vi "Uniform_spaced_data.vi"(1 "Desired Times":dbl[](array[numeric]) format="%.2f", 2 "Eng Value":dbl[](array[numeric]) format="%.2f", 3 "Current Times":dbl[](array[numeric]) format="%.2f") -> (0 "Eng Values out":dbl[](array[numeric]) format="%.2f")   [LabVIEW 2010]
uses:
  <vilib>/Analysis/NI_AALPro.lvlib
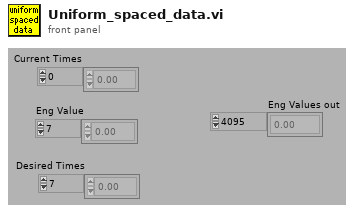
[diagram p1: front panel]
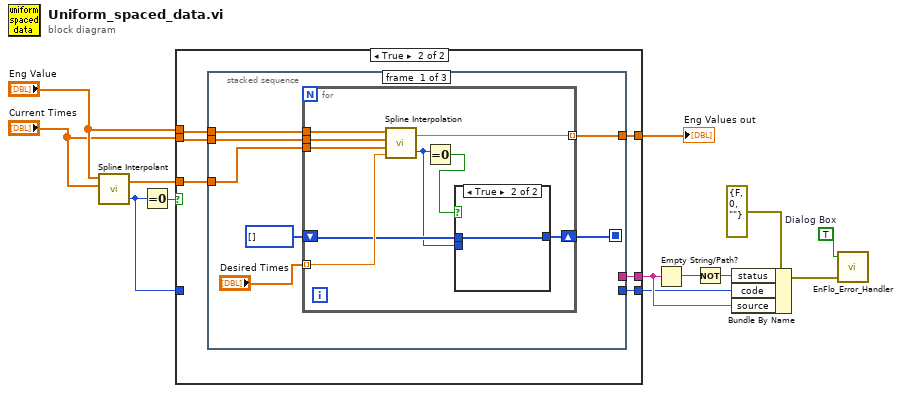
[diagram p0: block diagram]
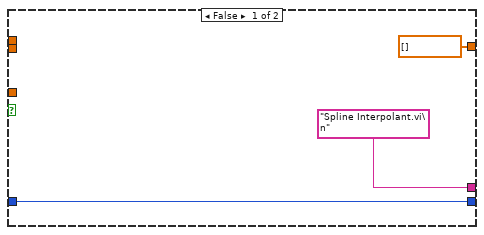
[diagram p2: hidden frame]
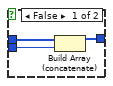
[diagram p3: hidden frame]
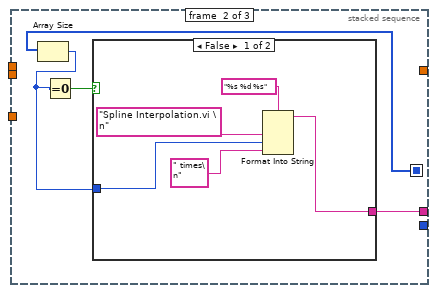
[diagram p4: hidden frame]
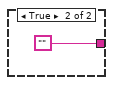
[diagram p5: hidden frame]
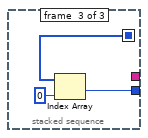
[diagram p6: hidden frame]
diagram:
  w2 = TRUE  # Dialog Box
  n1 = call <vilib>:"Spline Interpolant.vi"("X"="Current Times", "Y"="Eng Value") -> ("error"=w3:i32, "Interpolant"=w11:dbl[])  [unwired: 2 in]
  n2 = Equal To 0?(x=w3) -> (x = 0?=w8:bool)
  n3 = case shown="True" w8 {
    tunnel: "Eng Value" -> [_ w22]
    tunnel: "Current Times" -> [_ w21]
    tunnel: w11 -> [_ w20]
    tunnel: ["Spline Interpolant.vi\n" ("source") w19] -> w5
    tunnel: [w15 w18] -> w4
    tunnel: w3 -> [w15 _]
    tunnel: [dbl[] [] w17] -> w1
    frame False {
    }
    frame True {
      n4 = stacked-sequence {
        seq-local: [w24 _ _] -> [_ w43 w55]
        tunnel: w22 -> [w29 _ _]
        tunnel: w21 -> [w28 _ _]
        tunnel: w20 -> [w27 _ _]
        tunnel: [_ w44 _] -> w19
        tunnel: [_ _ w53] -> w18
        tunnel: [w23 _ _] -> w17
        frame #0 {
          n5 = for {
            tunnel: w29 -> [w38]
            tunnel: w28 -> [w37]
            tunnel: w27 -> [w36]
            tunnel: "Desired Times" -> [w35] mode=indexing
            shift-right: [w32] -> w24
            shift-left: i32[] [] -> [w33]
            tunnel: [w30] -> w23 mode=indexing
            n6 = call <vilib>:"Spline Interpolation.vi"("x value"=w35, "Interpolant"=w36, "X"=w37, "Y"=w38) -> ("error"=w31:i32, "interpolation value"=w30:dbl)
            n7 = Equal To 0?(x=w31) -> (x = 0?=w34:bool)
            n8 = case shown="True" w34 {
              tunnel: w33 -> [w41 w42]
              tunnel: [w40 w42] -> w32
              tunnel: w31 -> [w39 _]
              frame False {
                n9 = Build Array (concatenate)(w41, w39) -> (w40:i32[])
              }
              frame True {
              }
            }
          }
        }
        frame #1 {
          n10 = Array Size(array=w43) -> (size(s)=w45:i32)
          n11 = Equal To 0?(x=w45) -> (x = 0?=w46:bool)
          n12 = case shown="False" w46 {
            tunnel: w45 -> [w50 _]
            tunnel: [w47 ""] -> w44
            frame False {
              n13 = Format Into String(format string="%s %d %s" ("Format String"), "Spline Interpolation.vi \n" ("source"), w50, " times\n" ("source")) -> (resulting string=w47:string)  [unwired: 2 in, 1 out]
            }
            frame True {
            }
          }
        }
        frame #2 {
          n14 = Index Array(array=w55, index=0 ("Index")) -> (element=w53:i32)
        }
      }
    }
  }
  "Eng Values out" <- w1
  n15 = Empty String/Path?(string/path=w5) -> (empty?=w7:bool)
  n16 = Not(x=w7) -> (.not. x?=w6:bool)
  n17 = Bundle By Name(cluster=errorcluster {"status"=FALSE, "code"=0, "source"=""} ("error in (no error)"), "status"=w6, "code"=w4, "source"=w5) -> (w9:errorcluster)
  n18 = call "EnFlo_Error_Handler.vi"("error in (no error)"=w9, "Dialog Box (T)"=w2) -> ()  [unwired: 1 in, 3 out]
